vi "Set_Darkspec.vi"(8 "error in (no error)":errorcluster, 10 "Darkspec":T1(array[cluster]), 11 "Avantes in":refnum<class "Avantes.lvclass">) -> (0 "error out":errorcluster, 3 "Avantes out":refnum<class "Avantes.lvclass">)   [LabVIEW 2020, in "Avantes.lvclass"]
uses:
  <instrlib>/Classes/CCD/Avantes/Avantes.lvclass
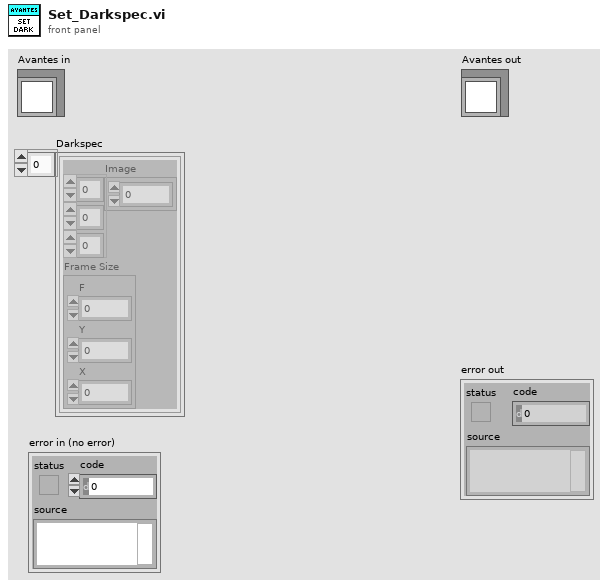
[diagram p1: front panel]
types:
  T1 = cluster{"Image":dbl[][][], "Frame Size":cluster{"F":i32, "Y":i32, "X":i32}}[]
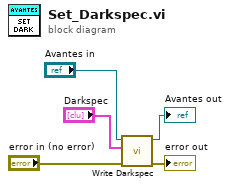
[diagram p0: block diagram]
diagram:
  n1 = call-dynamic "Write Darkspec.vi"("error in (no error)"="error in (no error)", "Darkspec"="Darkspec", "Avantes in"="Avantes in") -> ("error out"=→"error out":errorcluster, "Avantes out"=→"Avantes out":refnum<class "Avantes.lvclass">)  [unwired: 7 in]
